vi "Read Voltage and Output Frequency.vi"(0 "Analog Input Task In":refnum<k21>, 2 "V_PR Array In":dbl[](array[numeric]), 3 "Scale Frequency Array In":dbl[](array[numeric]), 5 "Error In":errorcluster) -> (11 "V_PR Array Element Out":dbl, 13 "Index Out":i32, 14 "Analog Input Task Out":refnum<k21>, 15 "V_PR Array Out":dbl[](array[numeric]), 16 "Scale Frequency Array Out":dbl[](array[numeric]), 17 "V_PR Reading Out":dbl, 18 "Frequency Out":dbl, 19 "Error Out":errorcluster)   [LabVIEW 2020]
doc: "Read Voltage and Output Frequency.vi reads the voltage across the photoresistor and converts it into a frequency from the Scale Frequency Array that corresponds to which two voltages contained in the V_PR Array it falls between."
uses:
  <vilib>/DAQmx/read.llb/DAQmx Read (Analog 1D DBL NChan 1Samp).vi
  <vilib>/DAQmx/miscellaneous.llb/DAQmx Fill In Error Info.vi
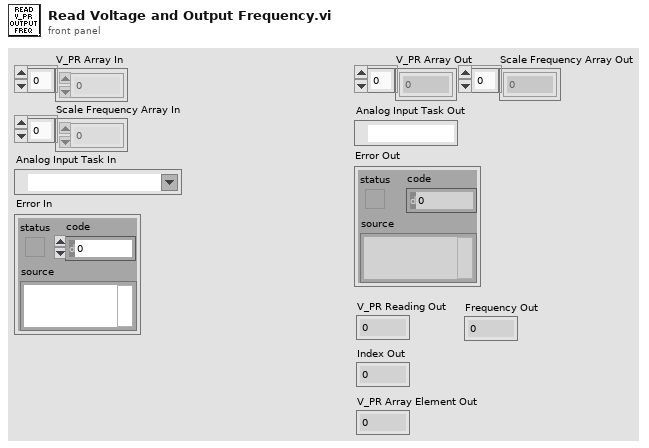
[diagram p1: front panel]
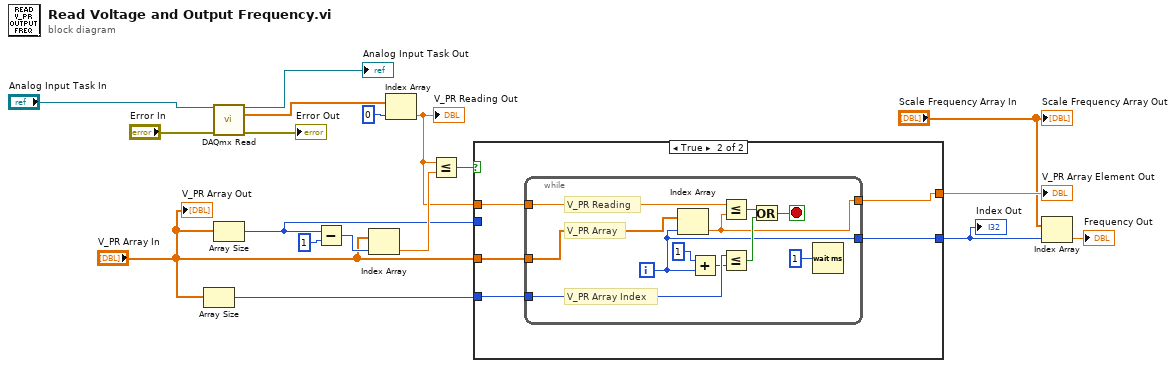
[diagram p0: block diagram]
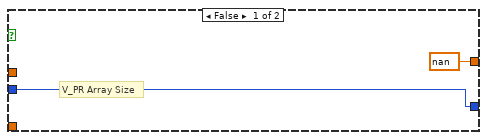
[diagram p2: hidden frame]
diagram:
  n1 = Array Size(array="V_PR Array In") -> (size(s)=w16:i32)
  n2 = call-poly <vilib>:"DAQmx Read.vi"("task/channels in"="Analog Input Task In", "error in"="Error In") -> ("task out"=→"Analog Input Task Out":refnum<k21>, "data"=w3:dbl[], "error out"=→"Error Out":errorcluster)  [unwired: 11 in]
  n3 = Array Size(array="V_PR Array In") -> (size(s)=w12:i32)
  n4 = Subtract(x=w12, y=1) -> (x-y=w10:i32)
  n5 = Index Array(array="V_PR Array In", index=w10) -> (element=w14:dbl)
  n6 = Index Array(array=w3, index=0) -> (element=w2:dbl)
  "V_PR Reading Out" <- w2
  n7 = Less Or Equal?(x=w2, y=w14) -> (x <= y?=w13:bool)
  n8 = case shown="True" w13 {
    tunnel: w16 -> [_ w25]
    tunnel: "V_PR Array In" -> [_ w24]
    tunnel: w2 -> [_ w23]
    tunnel: [nan w22] -> w15
    tunnel: [w20 w21] -> w9
    tunnel: w12 -> [w20 _]
    frame False {
      # "V_PR Array Size"
    }
    frame True {
      n9 = while {
        tunnel: w25 -> [w36]
        tunnel: w24 -> [w33]
        tunnel: w23 -> [w32]
        tunnel: [w28] -> w22
        tunnel: [w27] -> w21
        i -> [w27]
        stop <- w29 stop-if-true
        # "V_PR Array Index"
        # "V_PR Array"
        # "V_PR Reading"
        n10 = Index Array(array=w33, index=w27) -> (element=w28:dbl)
        n11 = Add(x=1, y=w27) -> (x+y=w34:i32)
        n12 = Less Or Equal?(x=w32, y=w28) -> (x <= y?=w30:bool)
        n13 = Less Or Equal?(x=w36, y=w34) -> (x <= y?=w31:bool)
        n14 = Or(x=w30, y=w31) -> (x .or. y?=w29:bool)
        n15 = Wait (ms)(milliseconds to wait=u32 1) -> ()  [unwired: 1 out]
      }
    }
  }
  "V_PR Array Element Out" <- w15
  "Index Out" <- w9
  n16 = Index Array(array="Scale Frequency Array In", index=w9) -> (element=→"Frequency Out":dbl)
  "V_PR Array Out" <- "V_PR Array In"
  "Scale Frequency Array Out" <- "Scale Frequency Array In"
